vi "SS_getMetaData.vi"(7 "error in":errorcluster, 10 "SweptSines":T1={"Log-Channel_select"=[FALSE, FALSE, FALSE, FALSE, FALSE, FALSE], "JSON Header"="", "SS-Params-Array"=[], "input_frequency_definitions"={"Amp"=0.0, "Ts"=0.0, "num_periodsMT"=[], "freqs_Hz"=[], "numAve_s"=[], "Nsamp_total"=[], "Nsettle_s"=[], "Ncollect_s"=[]}, "DAC-ADC primary 2"=0, "Channel-Names"=[], "num_chan"=0, "num-freqs"=0, "Input File (json)"=path "Z:/mpc-journal/sysID/FRF_data/x-axis_sines_info.json"} {"DAC-ADC primary 2" items=["DAC0/ADC0", "DAC1/ADC1", "DAC2/ADC2", "DAC3/ADC3", ""]}) -> (0 "error out":errorcluster, 2 "TsTicks":u32, 3 "SweptSines (out)":T1={"Log-Channel_select"=[FALSE, FALSE, FALSE, FALSE, FALSE, FALSE], "JSON Header"="", "SS-Params-Array"=[], "input_frequency_definitions"={"Amp"=0.0, "Ts"=0.0, "num_periodsMT"=[], "freqs_Hz"=[], "numAve_s"=[], "Nsamp_total"=[], "Nsettle_s"=[], "Ncollect_s"=[]}, "DAC-ADC primary 2"=0, "Channel-Names"=[], "num_chan"=0, "num-freqs"=0, "Input File (json)"=path "Z:/mpc-journal/sysID/FRF_data/x-axis_sines_info.json"} {"DAC-ADC primary 2" items=["DAC0/ADC0", "DAC1/ADC1", "DAC2/ADC2", "DAC3/ADC3", ""]})   [LabVIEW 2017]
uses:
  controls/SS_sin_params.ctl
  controls/SS_input_data_json.ctl
  controls/SS_SweptSines.ctl
  <vilib>/addons/_JKI.lib/Serialization/JSON/JKI JSON Serialization.lvlib
panel:
  in  "sin params":T3
  in  "sin params":T2
  out "Ts (from meta_data.csv)":dbl=1.0
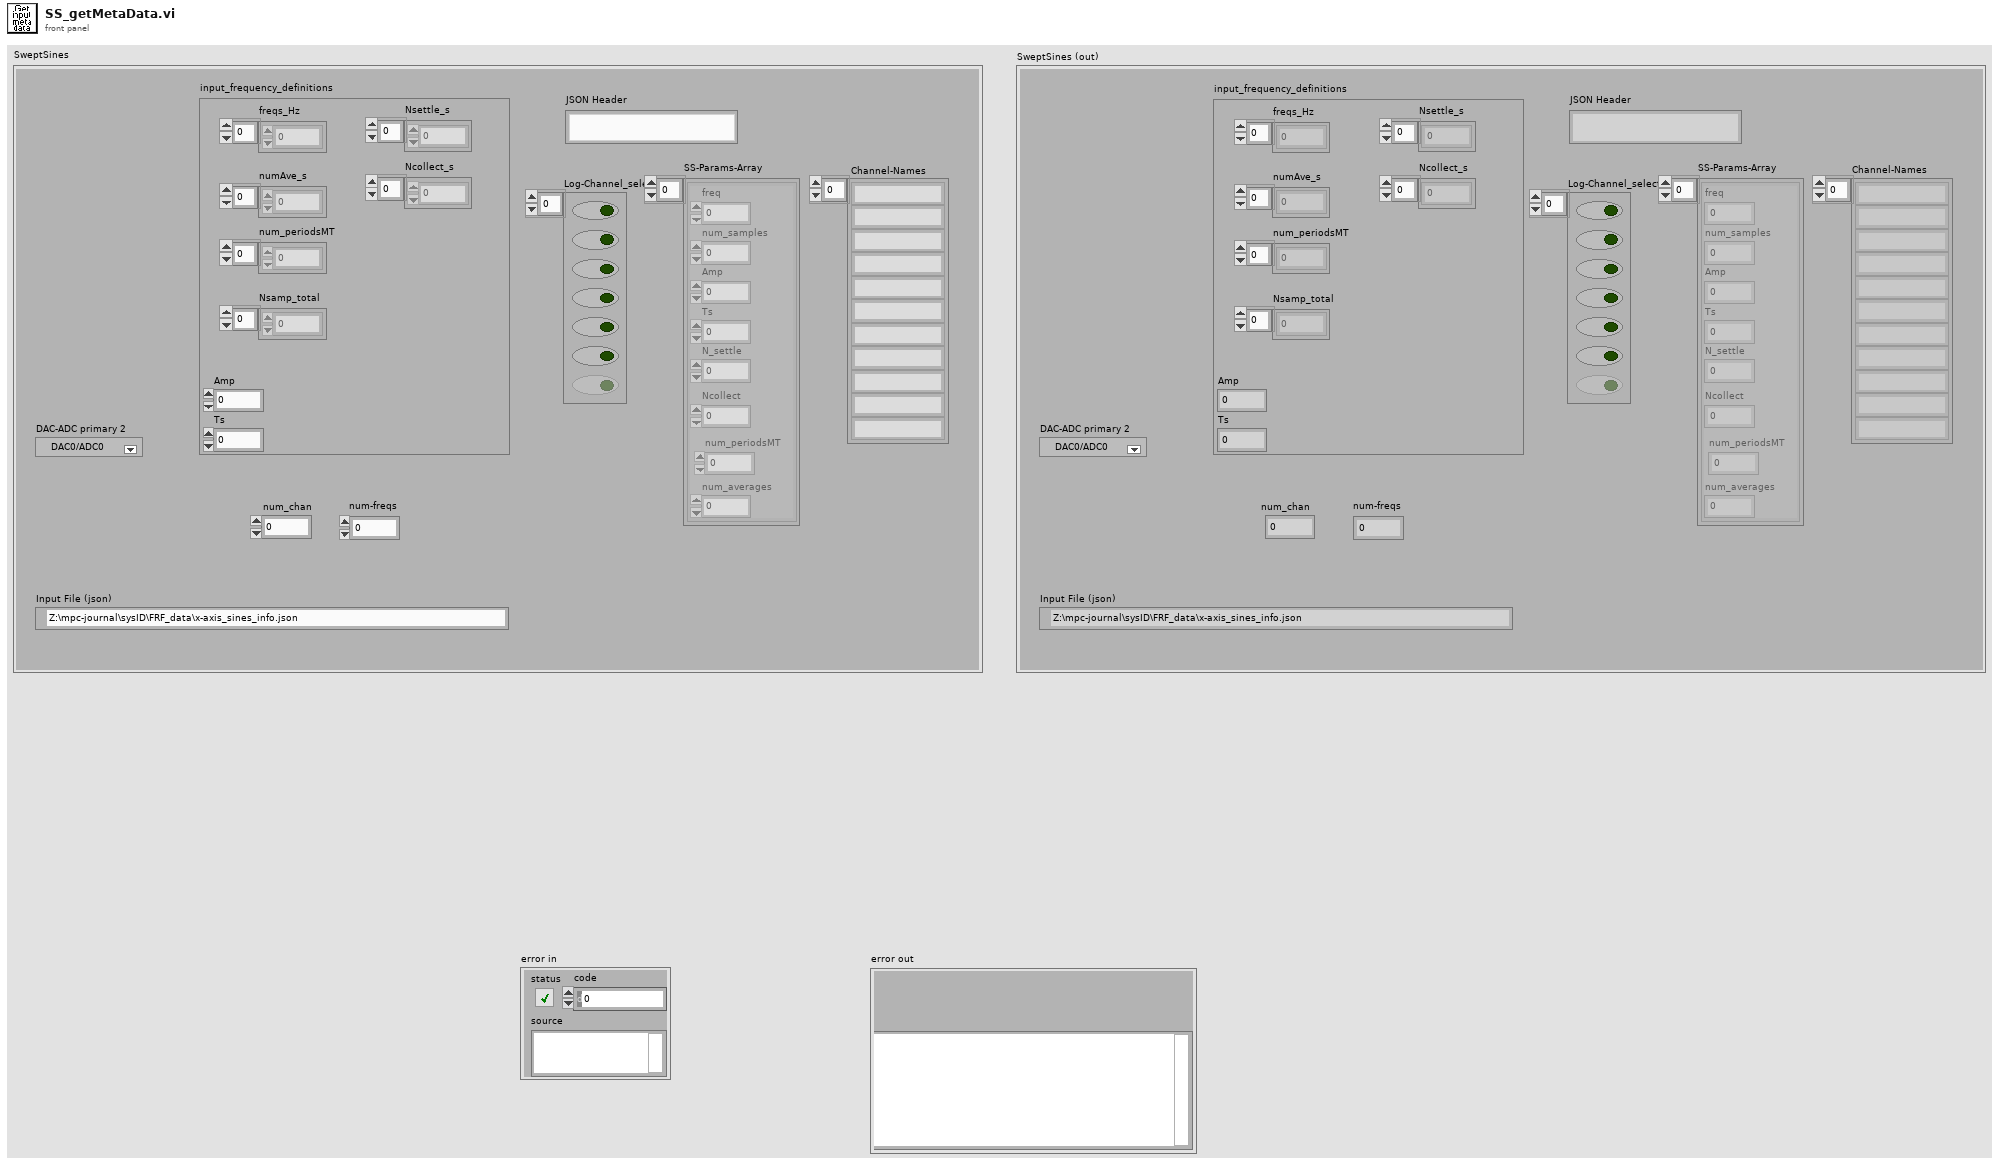
[diagram p1: front panel]
types:
  T1 = typedef "SS_SweptSines.ctl" = cluster{"Log-Channel_select":bool[], "JSON Header":string, "SS-Params-Array":T2[], "input_frequency_definitions":T3, "DAC-ADC primary 2":i16, "Channel-Names":string[], "num_chan":i32, "num-freqs":i32, "Input File (json)":path}
  T2 = typedef "SS_sin_params.ctl" = cluster{"freq":dbl, "num_samples":i32, "Amp":dbl, "Ts":dbl, "N_settle":u32, "Ncollect":i32, "num_periodsMT":i32, "num_averages":i32}
  T3 = typedef "SS_input_data_json.ctl" = cluster{"Amp":dbl, "Ts":dbl, "num_periodsMT":u32[], "freqs_Hz":dbl[], "numAve_s":i32[], "Nsamp_total":u32[], "Nsettle_s":u32[], "Ncollect_s":u32[]}
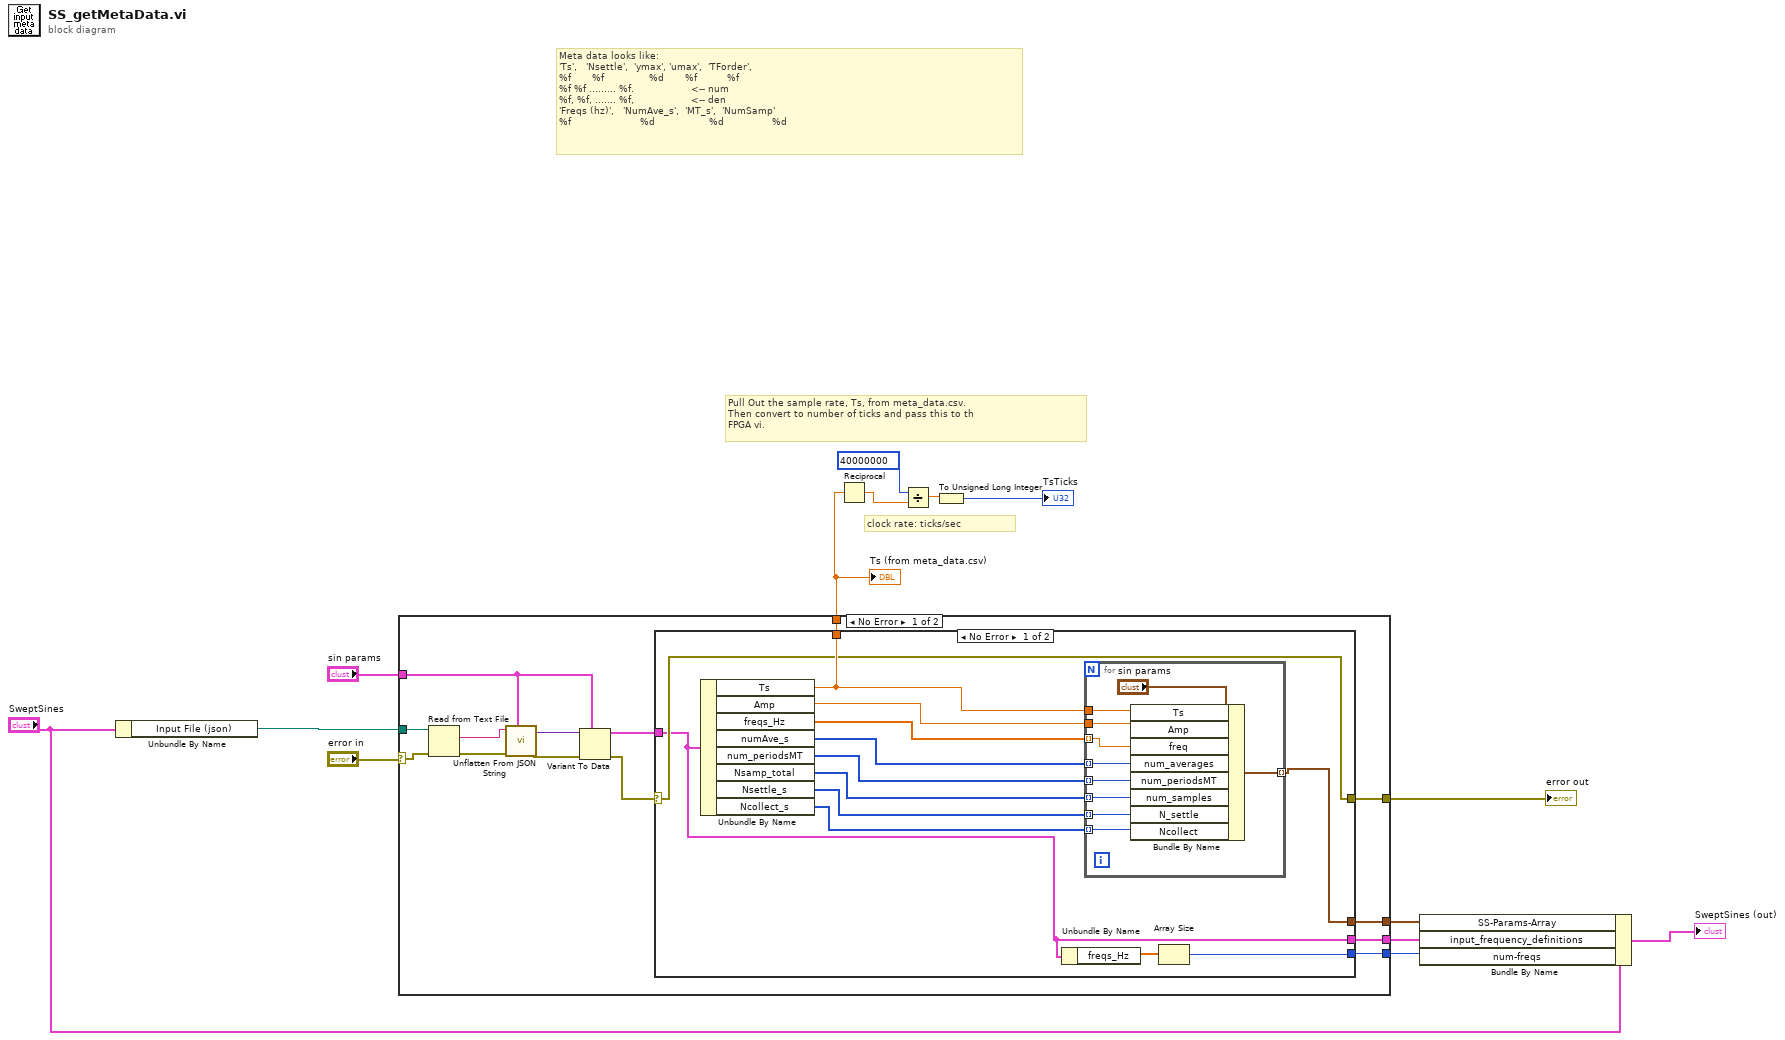
[diagram p0: block diagram]
diagram:
  # "Meta data looks like:\n'Ts',   'Nsettle',  'ymax', 'umax',  'TForder',\n%f       %f               %d       %f          %f\n%f %f ......... %f.                   <-- num\n%f, %f, ....... %f,                   <-- den      \n'Freqs (hz)',   'NumAve_s',  'MT_s',  'NumSamp'\n%f                       %d                  %d                %d"
  # "clock rate: ticks/sec"
  # "Pull Out the sample rate, Ts, from meta_data.csv.\nThen convert to number of ticks and pass this to th\nFPGA vi."
  n1 = Unbundle By Name("SweptSines") -> ("Input File (json)"=w8:path)
  n2 = case shown="No Error" "error in" {
    selector: "error in" -> [w16 w53]
    tunnel: "sin params" -> [w26 _]
    tunnel: [w23 _] -> w9
    tunnel: w8 -> [w22 _]
    tunnel: [w20 _] -> w6
    tunnel: [w18 _] -> w5
    tunnel: [w17 w53] -> w4
    tunnel: [w15 _] -> w1
    frame No Error {
      n3 = Read from Text File(file (use dialog)=w22, error in=w16) -> (text=w28:string, error out=w24:errorcluster)  [unwired: 2 in, 2 out]
      n4 = call <vilib>:"Unflatten From JSON String.vi"("Type and Defaults"=w26, "error in (no error)"=w24, "JSON String"=w28) -> ("error out"=w25:errorcluster, "Variant"=w27:variant)  [unwired: 7 in]
      n5 = Variant To Data(error in=w25, type=w26, Variant=w27) -> (data=w21:T3, error out=w19:errorcluster)
      n6 = case shown="No Error" w19 {
        selector: w19 -> [w32 w52]
        tunnel: [w34 _] -> w23
        tunnel: w21 -> [w31 _]
        tunnel: [w33 _] -> w20
        tunnel: [w31 _] -> w18
        tunnel: [w32 w52] -> w17
        tunnel: [w29 _] -> w15
        frame No Error {
          n7 = Unbundle By Name(w31) -> ("Ts"=w34:dbl, "Amp"=w41:dbl, "freqs_Hz"=w40:dbl[], "numAve_s"=w39:i32[], "num_periodsMT"=w38:u32[], "Nsamp_total"=w37:u32[], "Nsettle_s"=w36:u32[], "Ncollect_s"=w35:u32[])
          n8 = Unbundle By Name(w31) -> ("freqs_Hz"=w30:dbl[])
          n9 = for {
            tunnel: w40 -> [w44] mode=indexing
            tunnel: w37 -> [w51] mode=indexing
            tunnel: [w50] -> w33 mode=indexing
            tunnel: w41 -> [w45]
            tunnel: w34 -> [w46]
            tunnel: w36 -> [w47] mode=indexing
            tunnel: w35 -> [w48] mode=indexing
            tunnel: w38 -> [w43] mode=indexing
            tunnel: w39 -> [w42] mode=indexing
            n10 = Bundle By Name(cluster="sin params", "Ts"=w46, "Amp"=w45, "freq"=w44, "num_averages"=w42, "num_periodsMT"=w43, "num_samples"=w51, "N_settle"=w47, "Ncollect"=w48) -> (w50:T2)
          }
          n11 = Array Size(array=w30) -> (size(s)=w29:i32)
        }
        frame Error {
        }
      }
    }
    frame Error {
    }
  }
  "Ts (from meta_data.csv)" <- w9
  "error out" <- w4
  n12 = Reciprocal(x=w9) -> (1/x=w12:dbl)
  n13 = Divide(x=40000000, y=w12) -> (x/y=w14:dbl)
  n14 = To Unsigned Long Integer(number=w14) -> (unsigned 32bit integer=→"TsTicks":u32)
  n15 = Bundle By Name(cluster="SweptSines", "SS-Params-Array"=w6, "input_frequency_definitions"=w5, "num-freqs"=w1) -> (→"SweptSines (out)":T1)
